vi "Stop Core.vi"(10 "final error code":i32, 11 "State Machine in":refnum<class "State Machine.lvclass">) -> (3 "State Machine out":refnum<class "State Machine.lvclass">)   [LabVIEW 2024, in "State Machine.lvlib" / "State Machine.lvclass"]
doc: "<p>(<strong>Filename</strong>: <span class=\"dnl\">Actor Framework.lvlib:Actor.lvclass:Stop Core.vi</span>)</p>\n<p>Defines what the actor does before it stops. Use the <strong>final error code</strong> input to determine whether the actor shut down in response to an error.</p>\n<p>By default, this method passes the Stop message along to all <a href=\"nihelplauncher://docs/csh?context=lvcore_lvcomm_af_launch_nested_actor\">auto-stop nested actors</a>. A descendant class may override this method to define additional behavior, such as shutting down any processes the actor initiated in its override of the <a href=\"nihelplauncher://docs/csh?context=lvcore_lvcomm_af_actor_core\">Actor Core</a> method.</p>"
uses:
  State Machine.lvclass
  State Machine.lvclass/State Machine.ctl
  <vilib>/ActorFramework/Actor/Actor.lvclass
  Context/Context/Context.lvclass
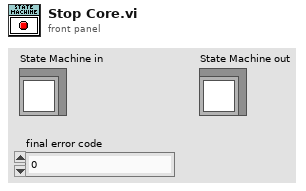
[diagram p1: front panel]
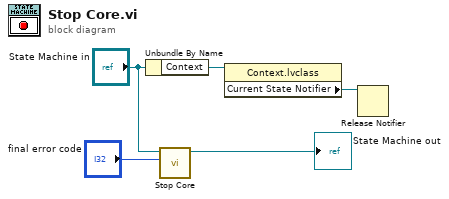
[diagram p0: block diagram]
diagram:
  n1 = Unbundle By Name("State Machine in") -> ("Context"=w3:refnum<class "Context.lvclass">)
  n2 = call-parent "Stop Core.vi"("final error code"="final error code", "Actor in"="State Machine in") -> ("Actor out"=→"State Machine out":refnum<class "State Machine.lvclass">)  [unwired: 9 in]
  n3 = property class="Context.lvclass"(reference=w3) -> ("Current State Notifier"=w2:refnum<notifier>)  [unwired: 1 in, 2 out]
  n4 = Release Notifier(notifier=w2) -> ()  [unwired: 2 in, 3 out]
